vi "Shutdown Sink.vi"(8 "error in (no error)":errorcluster, 11 "Log Sink":refnum<data-value>) -> (0 "error out":errorcluster)   [LabVIEW 2017, in "Composed Log.lvlib" / "Log Sink.lvclass"]
uses:
  Log Sink.lvclass
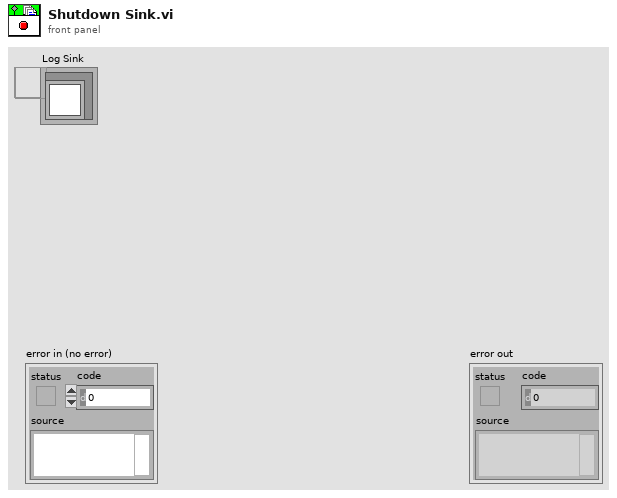
[diagram p1: front panel]
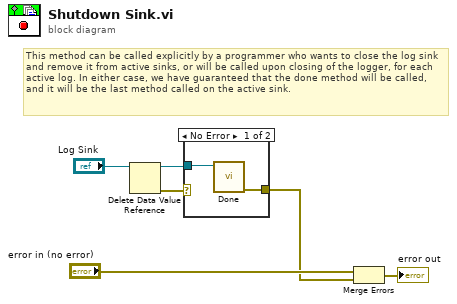
[diagram p0: block diagram]
diagram:
  # "This method can be called explicitly by a programmer who wants to close the log sink and remove it from active sinks, or will be called upon closing of the logger, for each active log. In either case, we have guaranteed that the done method will be called, and it will be the last method called on the active sink."
  n1 = Delete Data Value Reference(data value reference="Log Sink") -> (data value=w2:refnum<class "Log Sink.lvclass">, error out=w3:errorcluster)  [unwired: 1 in]
  n2 = case shown="No Error" w3 {
    tunnel: w2 -> [w8 _]
    tunnel: [w7 _] -> w1
    frame No Error {
      n3 = call-dynamic "Done.vi"("Log Sink in"=w8) -> ("error out"=w7:errorcluster)  [unwired: 10 in]
    }
    frame Error {
    }
  }
  n4 = Merge Errors("error in (no error)", w1) -> (→"error out":errorcluster)
